vi "Discover roboRIO.vi"(8 "error in (no error)":errorcluster, 11 "roboRIO Connection Information in":T1) -> (0 "error out":errorcluster, 3 "roboRIO Connection Information out":T1)   [LabVIEW 2018, in "Personalities Tool.lvlib"]
doc: "Use this VI to discover a roboRIO connected to the computer.\nThis VI does not look for the personality and will return an invalid one for the roboRIO."
uses:
  Personalities Tool.lvlib
  Controls/roboRIO Connection Information.ctl
  Controls/Personality Type.ctl
  <vilib>/nisyscfg/Close (System).vi
  <vilib>/Utility/config.llb/Read Key (String).vi
  <vilib>/nisyscfg/nisyscfg.lvlib
  <resource>/objmgr/nisysapi.rc
  <vilib>/FTP/NI_FTP.lvlib
  <vilib>/Utility/config.llb/NI_LVConfig.lvlib
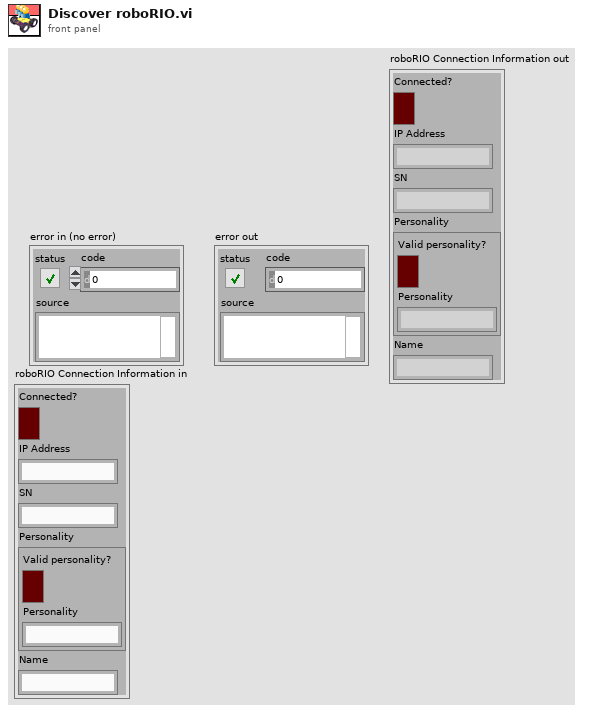
[diagram p1: front panel]
types:
  T1 = typedef "Personalities Tool.lvlib/roboRIO Connection Information.ctl" = cluster{"Connected?":bool, "IP Address":string, "SN":string, "Personality":T2, "Name":string}
  T2 = typedef "Personalities Tool.lvlib/Personality Type.ctl" = cluster{"Valid personality?":bool, "Personality":string}
  T3 = typedef "NI_LVConfig.lvlib/Config Data RefNum.ctl" = refnum<k1>
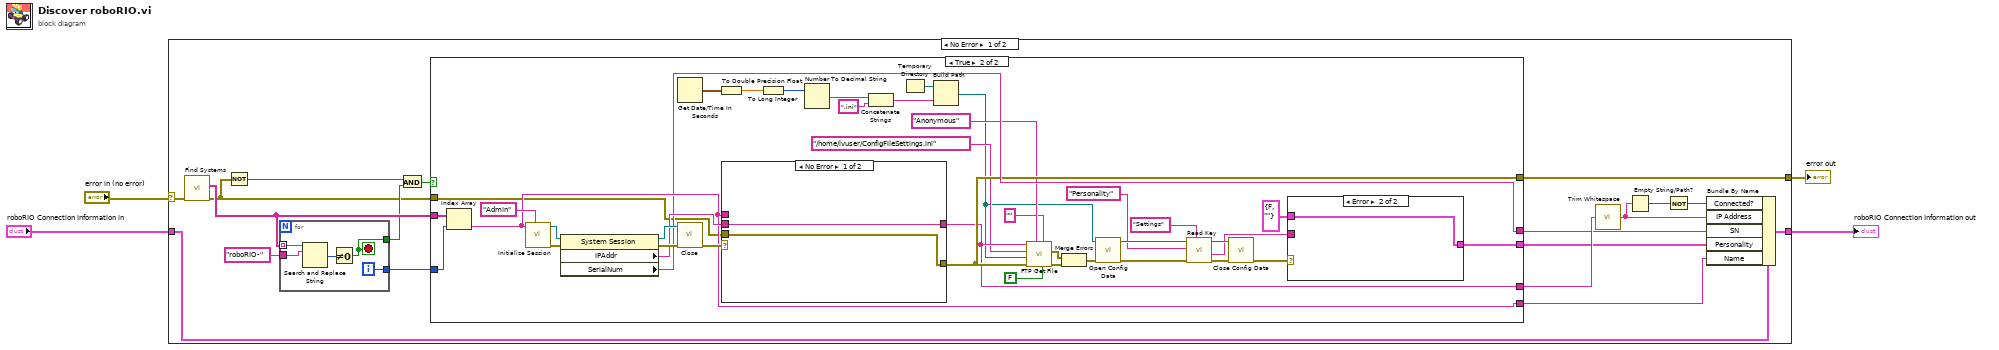
[diagram p0: block diagram]
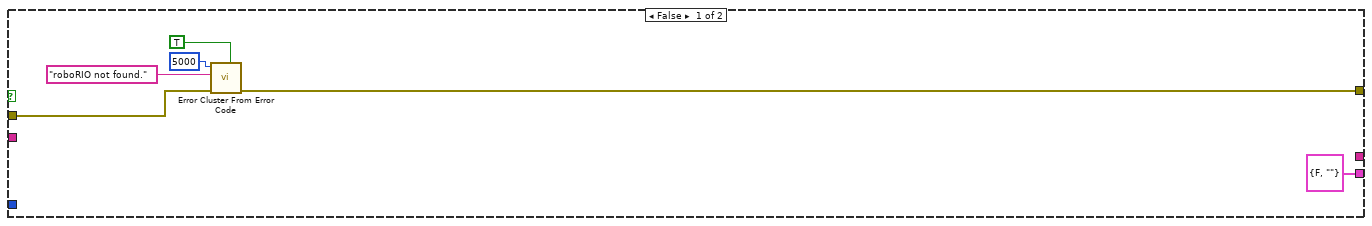
[diagram p2: hidden frame]
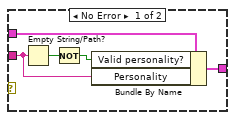
[diagram p3: hidden frame]
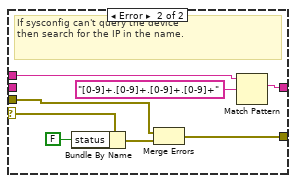
[diagram p4: hidden frame]
diagram:
  n1 = case shown="No Error" "error in (no error)" {
    selector: "error in (no error)" -> [w20 w90]
    tunnel: [w22 w90] -> w4
    tunnel: "roboRIO Connection Information in" -> [w13 w89]
    tunnel: [w12 w89] -> w1
    frame No Error {
      n2 = call <vilib>:"Find Systems.vi"("error in (no error)"=w20) -> ("error out"=w7:errorcluster, "Detected Systems"=w18:string[])  [unwired: 8 in, 1 out]
      n3 = Not(x=w7) -> (.not. x?=w14:bool)
      n4 = for {
        tunnel: w18 -> [w88] mode=indexing
        tunnel: "roboRIO-" ("string") -> [w87]
        tunnel: [w85] -> w17
        tunnel: [w84] -> w16
        i -> [w84]
        stop <- w85 stop-if-true
        n5 = Search and Replace String(input string=w88, search string=w87) -> (number of replacements=w86:i32)  [unwired: 6 in, 3 out]
        n6 = Not Equal To 0?(x=w86) -> (x != 0?=w85:bool)
      }
      n7 = And(x=w14, y=w17) -> (x .and. y?=w15:bool)
      n8 = case shown="True" w15 {
        tunnel: w18 -> [_ w62]
        tunnel: w16 -> [_ w61]
        tunnel: [_ w58] -> w8
        tunnel: [_ w54] -> w21
        tunnel: [w25 w55] -> w22
        tunnel: [_ w57] -> w11
        tunnel: w7 -> [w24 w56]
        tunnel: [T2 {"Valid personality?"=FALSE, "Personality"=""} ("Personality") w35] -> w5
        frame False {
          n9 = call <vilib>:"Error Cluster From Error Code.vi"("is warning? (False)"=TRUE, "error in (no error)"=w24, "error message (\"\")"="roboRIO not found." ("error message (\"\")"), "error code (0)"=5000) -> ("error out"=w25:errorcluster)  [unwired: 5 in]
        }
        frame True {
          n10 = Index Array(array=w62, index=w61) -> (element=w58:string)
          n11 = call <vilib>:"Initialize Session.vi"("User Name"="Admin", "Target (localhost)"=w58) -> ("error out"=w66:errorcluster, "Session out"=w67:refnum<k21>)  [unwired: 8 in]
          n12 = property class="System Session"(reference=w67, error in=w66) -> (reference out=w65:refnum<k21>, error out=w64:errorcluster, "IPAddr"=w59:string, "SerialNum"=w57:string)
          n13 = Get Date/Time In Seconds() -> (seconds since 1Jan1904=w30:timestamp)
          n14 = call-poly <vilib>:"Close.vi"("error in (no error)"=w64, "Session in"=w65) -> ("error out"=w60:errorcluster)  [unwired: 9 in]
          n15 = To Double Precision Float(number=w30) -> (double precision float=w29:dbl)
          n16 = case shown="No Error" w60 {
            selector: w60 -> [_ w78]
            tunnel: [w75 w81] -> w54
            tunnel: w59 -> [w75 _]
            tunnel: w58 -> [_ w83]
            tunnel: w56 -> [w74 w80]
            tunnel: [w74 w79] -> w55
            frame No Error {
            }
            frame Error {
              # "If sysconfig can't query the device\nthen search for the IP in the name."
              n17 = Bundle By Name(cluster=w78, "status"=FALSE) -> (w77:errorcluster)
              n18 = Merge Errors(w80, w77) -> (w79:errorcluster)
              n19 = Match Pattern(string=w83, regular expression="[0-9]+.[0-9]+.[0-9]+.[0-9]+") -> (match substring=w81:string)  [unwired: 1 in, 3 out]
            }
          }
          n20 = To Long Integer(number=w29) -> (32bit integer=w51:i32)
          n21 = Number To Decimal String(number=w51) -> (decimal integer string=w50:string)  [unwired: 1 in]
          n22 = Concatenate Strings(w50, ".ini" ("string")) -> (w49:string)
          n23 = Temporary Directory() -> (w52:path)
          n24 = Build Path(base path=w52, name or relative path=w49) -> (appended path=w38:path)
          n25 = call <vilib>:"FTP Get File.vi"("active (T)"=FALSE, "password"="" ("user"), "user"="Anonymous", "error in (no error)"=w55, "local path"=w38, "remote path"="/home/lvuser/ConfigFileSettings.ini", "host"=w54) -> ("error out"=w44:errorcluster, "file error"=w45:errorcluster)  [unwired: 3 in]
          n26 = Merge Errors(w45, w44) -> (w43:errorcluster)
          n27 = call <vilib>:"Open Config Data.vi"("error in (no error)"=w43, "configuration file path"=w38) -> ("error out"=w41:errorcluster, "refnum"=w42:T3)  [unwired: 7 in, 1 out]
          n28 = call-poly <vilib>:"Read Key.vi"("section"="Settings", "error in (no error)"=w41, "key"="Personality", "refnum"=w42) -> ("error out"=w39:errorcluster, "value"=w34:string, "refnum out"=w40:T3)  [unwired: 4 in, 1 out]
          n29 = call <vilib>:"Close Config Data.vi"("error in (no error)"=w39, "refnum"=w40) -> ("error out"=w37:errorcluster)  [unwired: 8 in, 1 out]
          n30 = case shown="Error" w37 {
            tunnel: T2 {"Valid personality?"=FALSE, "Personality"=""} ("Personality") -> [w70 w73]
            tunnel: [w68 w73] -> w35
            tunnel: w34 -> [w71 _]
            frame No Error {
              n31 = Empty String/Path?(string/path=w71) -> (empty?=w72:bool)
              n32 = Not(x=w72) -> (.not. x?=w69:bool)
              n33 = Bundle By Name(cluster=w70, "Valid personality?"=w69, "Personality"=w71) -> (w68:T2)
            }
            frame Error {
            }
          }
        }
      }
      n34 = call <vilib>:"Trim Whitespace.vi"("string"=w21) -> ("trimmed string"=w9:string)  [unwired: 1 in]
      n35 = Empty String/Path?(string/path=w9) -> (empty?=w10:bool)
      n36 = Not(x=w10) -> (.not. x?=w6:bool)
      n37 = Bundle By Name(cluster=w13, "Connected?"=w6, "IP Address"=w9, "SN"=w11, "Personality"=w5, "Name"=w8) -> (w12:T1)
    }
    frame Error {
    }
  }
  "error out" <- w4
  "roboRIO Connection Information out" <- w1
